vi "Agilent SNA Set Stimulus.vi"(5 "Stimulus":T4={"Use Instrument Settings"=FALSE, "Blank Frequencies"=FALSE, "Sweep Type"=enum."Linear", "Sweep"={"Fstart"=500.0, "Fstop"=1500.0, "Units"=enum."MHz", "Points"=201}, "Power (dBm)"=999.0, "IFBW (Hz)"=-1.0, "Sweep Time (s)"=-1.0, "Calibration"={"State"=FALSE, "String"=""}} {"Sweep Time (s)" format="%.3g"}, 6 "Set Stimulus? (T)":bool=TRUE, 7 "Agilent SNA":T7, 8 "error in (no error)":errorcluster, 9 "Channel":i8=1 min=1 max=99 step=1, 10 "Sorted Measurements":cluster{"Measurements":T1[]}[](array[cluster]) {"Measurements"."Traces"."Parameter"."Stimulus Port" min=1 step=1; "Measurements"."Traces"."Parameter"."Response Port" min=1 step=1}, 11 "VISA Resource Names":T3) -> (0 "error out":errorcluster {"code" format="%.0x"}, 3 "dup VISA Resource Names":T3)   [LabVIEW 2011]
uses:
  TypeDefs/Agilent SNA VISA.ctl
  TypeDefs/Agilent SNA Instrument Info.ctl
  tests/S Parameter/TypeDefs/SP Stimulus Parameters.ctl
  tests/S Parameter/TypeDefs/SP Frequency Units.ctl
  tests/S Parameter/TypeDefs/SP Calibration State.ctl
  TypeDefs/Agilent SNA Measurements.ctl
  tests/S Parameter/TypeDefs/SP Parameter.ctl
  TypeDefs/Agilent SNA Measurement.ctl
  TypeDefs/Agilent SNA Message Mode.ctl
  TypeDefs/Agilent SNA External Trigger Mode.ctl
  TypeDefs/Agilent SNA Sweep Type.ctl
  TypeDefs/Agilent SNA Trigger Mode.ctl
panel:
  in  "Case Constant\n(See Context Help)":bool
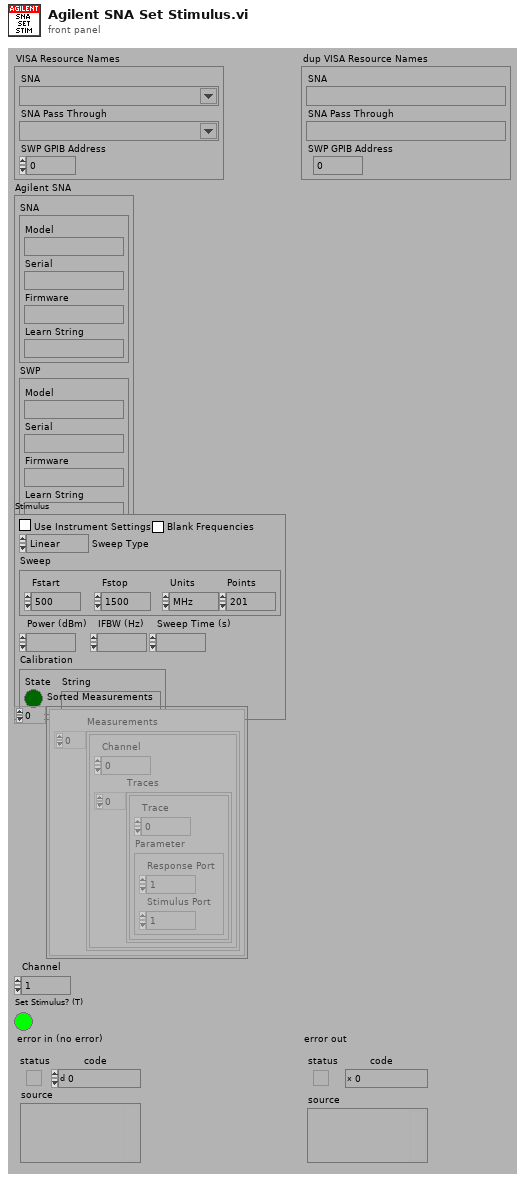
[diagram p1: front panel]
types:
  T1 = typedef "Agilent SNA Measurements.ctl" = cluster{"Channel":i8, "Traces":cluster{"Trace":i8, "Parameter":T2}[]}
  T2 = typedef "SP Parameter.ctl" = cluster{"Stimulus Port":i8, "Response Port":i8}
  T3 = typedef "Agilent SNA VISA.ctl" = cluster{"SNA":refnum<visa-resource-name>, "SNA Pass Through":refnum<visa-resource-name>, "SWP GPIB Address":i32}
  T4 = typedef "SP Stimulus Parameters.ctl" = cluster{"Use Instrument Settings":bool, "Blank Frequencies":bool, "Sweep Type":enum32{"Linear", "Logarithmic", "List", "Power", "CW"}, "Sweep":cluster{"Fstart":dbl, "Fstop":dbl, "Units":T5, "Points":i32}, "Power (dBm)":dbl, "IFBW (Hz)":dbl, "Sweep Time (s)":dbl, "Calibration":T6}
  T5 = typedef "SP Frequency Units.ctl" = enum16{"Hz", "kHz", "MHz", "GHz", "Points"}
  T6 = typedef "SP Calibration State.ctl" = cluster{"State":bool, "String":string}
  T7 = typedef "Agilent SNA Instrument Info.ctl" = cluster{"SNA":cluster{"Model":string, "Serial":string, "Firmware":string, "Learn String":string}, "SWP":cluster{"Model":string, "Serial":string, "Firmware":string, "Learn String":string}}
  T8 = typedef "Agilent SNA Message Mode.ctl" = enum16{"On", "Off"}
  T9 = typedef "Agilent SNA Measurement.ctl" = enum32{"SXX", "A", "B", "C", "R", "A/B", "A/C", "A/R", "B/A", "B/C", "B/R", "C/A", "C/B", "C/R", "R/A", "R/B", "R/C", "Analog In - Aux In"}
  T10 = typedef "Agilent SNA External Trigger Mode.ctl" = enum16{"Internal", "External", "Single/Bus"}
  T11 = typedef "Agilent SNA Sweep Type.ctl" = enum32{"Linear Sweep", "CW Time Sweep", "Frequency List"}
  T12 = typedef "Agilent SNA Trigger Mode.ctl" = enum16{"Continuous", "Hold", "Single"}
  T13 = enum32{"Linear", "Logarithmic", "List", "Power", "CW"}
  T14 = cluster{"Converted Frequency":dbl, "Converted Frequency":dbl}
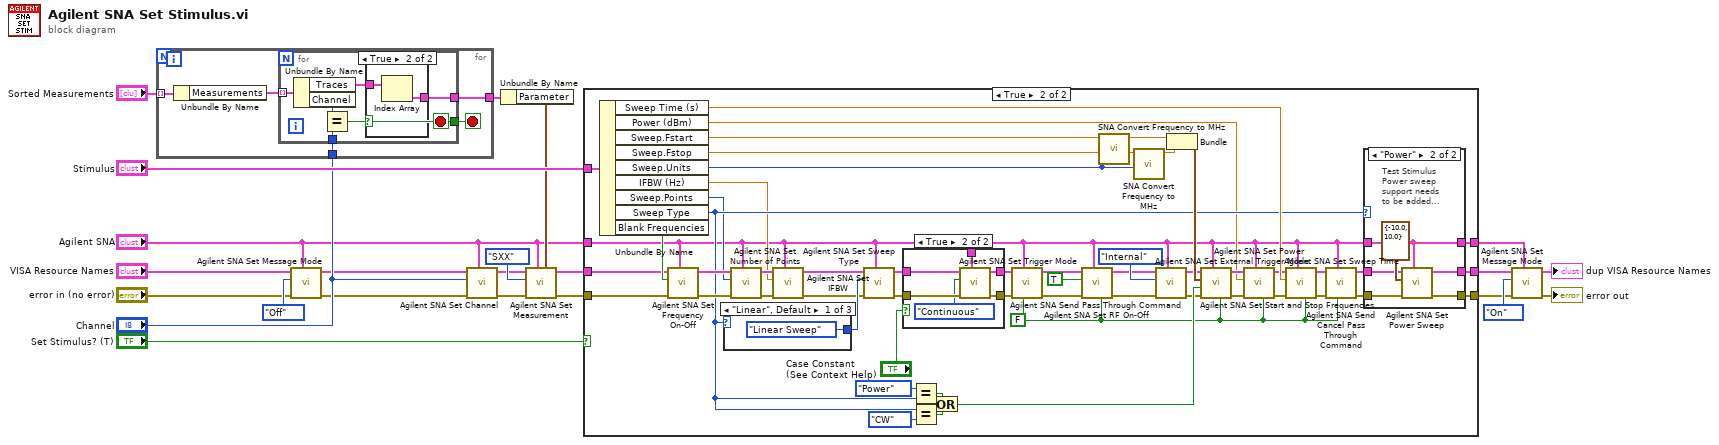
[diagram p0: block diagram]
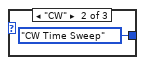
[diagram p4: hidden frame]
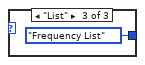
[diagram p5: hidden frame]
diagram:
  n1 = for {
    tunnel: "Sorted Measurements" -> [w28] mode=indexing
    tunnel: "Channel" -> [w26]
    tunnel: [w25] -> w14
    stop <- w24 stop-if-true
    n2 = Unbundle By Name(w28) -> ("Measurements"=w27:T1[])
    n3 = for {
      tunnel: w27 -> [w34] mode=indexing
      tunnel: w26 -> [w31]
      tunnel: [w30] -> w25
      tunnel: [w29] -> w24
      stop <- w29 stop-if-true
      n4 = Unbundle By Name(w34) -> ("Traces"=w32:cluster{"Trace":i8, "Parameter":T2}[], "Channel"=w33:i8)
      n5 = Equal?(x=w33, y=w31) -> (x = y?=w29:bool)
      n6 = case shown="True" w29 {
        tunnel: w32 -> [_ w36]
        tunnel: [_ w35] -> w30
        frame False {
        }
        frame True {
          n7 = Index Array(array=w36) -> (element=w35:cluster{"Trace":i8, "Parameter":T2})  [unwired: 1 in]
        }
      }
    }
  }
  n8 = call "Agilent SNA Set Message Mode.vi"("Agilent SNA & SWP"="Agilent SNA", "error in (no error)"="error in (no error)", "Message Mode"=Agilent_SNA_Message_Mode."Off", "VISA Resource Names"="VISA Resource Names") -> ("error out"=w3:errorcluster, "dup VISA Resource Names"=w4:T3)  [unwired: 6 out]
  n9 = call "Agilent SNA Set Channel.vi"("Agilent SNA & SWP"="Agilent SNA", "error in (no error)"=w3, "Channel"="Channel", "VISA Resource Names"=w4) -> ("error out"=w19:errorcluster, "dup VISA Resource Names"=w20:T3)  [unwired: 6 out]
  n10 = Unbundle By Name(w14) -> ("Parameter"=w13:T2)
  n11 = call "Agilent SNA Set Measurement.vi"("Parameter"=w13, "Agilent SNA & SWP"="Agilent SNA", "error in (no error)"=w19, "Measurement (SXX)"=Agilent_SNA_Measurement."SXX" ("Measurement (S11 - A/R)"), "VISA Resource Names"=w20) -> ("error out"=w18:errorcluster, "dup VISA Resource Names"=w17:T3)  [unwired: 3 in, 2 out]
  n12 = case shown="True" "Set Stimulus? (T)" {
    tunnel: "Stimulus" -> [_ w92]
    tunnel: w18 -> [w39 w76]
    tunnel: w17 -> [w38 w77]
    tunnel: [w39 w63] -> w8
    tunnel: [w38 w64] -> w7
    tunnel: "Agilent SNA" -> [w37 w48]
    tunnel: [w37 w40] -> w1
    frame False {
    }
    frame True {
      w47 = FALSE ("SCPI? (F)")
      n13 = Unbundle By Name(w92) -> ("Sweep Time (s)"=w91:dbl, "Power (dBm)"=w60:dbl, "Sweep.Fstart"=w59:dbl, "Sweep.Fstop"=w58:dbl, "Sweep.Units"=w57:T5, "IFBW (Hz)"=w67:dbl, "Sweep.Points"=w68:i32, "Sweep Type"=w69:T13, "Blank Frequencies"=w83:bool)
      n14 = call "Agilent SNA Set Frequency On-Off.vi"("Agilent SNA & SWP"=w48, "error in (no error)"=w76, "Blank Frequencies (F)"=w83, "VISA Resource Names"=w77) -> ("error out"=w70:errorcluster, "dup VISA Resource Names"=w71:T3)  [unwired: 6 out]
      n15 = case shown="\"Linear\", Default" w69 {
        tunnel: [Agilent_SNA_Sweep_Type."Linear Sweep" ("Sweep Type") Agilent_SNA_Sweep_Type."CW Time Sweep" ("Sweep Type") Agilent_SNA_Sweep_Type."Frequency List" ("Sweep Type")] -> w80
        frame "Linear", Default {
        }
        frame "CW" {
        }
        frame "List" {
        }
      }
      n16 = call "Agilent SNA Set Number of Points.vi"("Agilent SNA & SWP"=w48, "error in (no error)"=w70, "Number Points"=w68, "VISA Resource Names"=w71) -> ("error out"=w74:errorcluster, "dup VISA Resource Names"=w75:T3)  [unwired: 1 in, 5 out]
      n17 = call "Agilent SNA Set IFBW.vi"("Agilent SNA & SWP"=w48, "error in (no error)"=w74, "IFBW, Hz (1000)"=w67, "VISA Resource Names"=w75) -> ("error out"=w73:errorcluster, "dup VISA Resource Names"=w72:T3)  [unwired: 1 in, 5 out]
      n18 = call "Agilent SNA Set Sweep Type.vi"("Agilent SNA & SWP"=w48, "error in (no error)"=w73, "Sweep Type"=w80, "VISA Resource Names"=w72) -> ("error out"=w55:errorcluster, "dup VISA Resource Names"=w56:T3)  [unwired: 1 in, 5 out]
      n19 = case shown="True" "Case Constant\n(See Context Help)" {
        tunnel: [w97 w100] -> w45
        tunnel: [w96 w101] -> w46
        tunnel: w55 -> [w97 w103]
        tunnel: w56 -> [w96 w102]
        tunnel: w48 -> [_ w98]
        frame False {
        }
        frame True {
          n20 = call "Agilent SNA Set Trigger Mode.vi"("Agilent SNA & SWP"=w98, "error in (no error)"=w103, "Trigger Mode"=Agilent_SNA_Trigger_Mode."Continuous", "VISA Resource Names"=w102) -> ("error out"=w100:errorcluster, "dup VISA Resource Names"=w101:T3)  [unwired: 1 in, 5 out]
        }
      }
      n21 = Equal?(x=enum32{"Linear", "Log", "List", "Power", "CW"}."Power" ("Sweep Type"), y=w69) -> (x = y?=w88:bool)
      n22 = Equal?(x=w69, y=enum32{"Linear", "Log", "List", "Power", "CW"}."CW" ("Sweep Type")) -> (x = y?=w87:bool)
      n23 = Or(x=w88, y=w87) -> (x .or. y?=w84:bool)
      n24 = call "Agilent SNA Send Pass Through Command.vi"("SCPI? (F)"=w47, "Agilent SNA & SWP"=w48, "error in (no error)"=w45, "VISA Resource Names"=w46) -> ("error out"=w54:errorcluster, "dup VISA Resource Names"=w53:T3)  [unwired: 6 out]
      n25 = call "Agilent SNA Set RF On-Off.vi"("Passthrough (T)"=w47, "Agilent SNA & SWP"=w48, "error in (no error)"=w54, "RF On (T)"=TRUE, "VISA Resource Names"=w53) -> ("error out"=w41:errorcluster, "dup VISA Resource Names"=w42:T3)  [unwired: 5 out]
      n26 = call "SNA Convert Frequency to MHz.vi"("Units"=w57, "Frequency"=w59) -> ("Converted Frequency"=w82:dbl)  [unwired: 9 out]
      n27 = call "SNA Convert Frequency to MHz.vi"("Units"=w57, "Frequency"=w58) -> ("Converted Frequency"=w81:dbl)  [unwired: 9 out]
      n28 = call "Agilent SNA Set External Trigger Mode.vi"("Agilent SNA & SWP"=w48, "error in (no error)"=w41, "Ext. Trigger Mode"=Agilent_SNA_External_Trigger_Mode."Internal", "VISA Resource Names"=w42) -> ("error out"=w44:errorcluster, "dup VISA Resource Names"=w43:T3)  [unwired: 1 in, 5 out]
      n29 = Bundle("Converted Frequency"=w82, "Converted Frequency"=w81) -> (w89:T14)  [unwired: 1 out]
      n30 = call "Agilent SNA Set Start and Stop Frequencies.vi"("Passthrough (T)"=w47, "Agilent SNA & SWP"=w48, "error in (no error)"=w44, "CW? (f)"=w84, "Start/Stop Freqs, MHz"=w89, "VISA Resource Names"=w43) -> ("error out"=w62:errorcluster, "dup VISA Resource Names"=w61:T3)  [unwired: 1 in, 3 out]
      n31 = call "Agilent SNA Set Power.vi"("Passthrough (T)"=w47, "Agilent SNA & SWP"=w48, "error in (no error)"=w62, "Source Power, dBm (0.0)"=w60, "VISA Resource Names"=w61) -> ("error out"=w65:errorcluster, "dup VISA Resource Names"=w66:T3)  [unwired: 1 in, 4 out]
      n32 = call "Agilent SNA Set Sweep Time.vi"("Passthrough (T)"=w47, "Agilent SNA & SWP"=w48, "error in (no error)"=w65, "Sweep Time, s (-1: Auto)"=w91, "VISA Resource Names"=w66) -> ("error out"=w51:errorcluster, "dup VISA Resource Names"=w52:T3)  [unwired: 1 in, 4 out]
      n33 = call "Agilent SNA Send Cancel Pass Through Command.vi"("SCPI? (F)"=w47, "Agilent SNA & SWP"=w48, "error in (no error)"=w51, "VISA Resource Names"=w52) -> ("error out"=w50:errorcluster, "dup VISA Resource Names"=w49:T3)  [unwired: 6 out]
      n34 = case shown="\"Power\"" w69 {
        tunnel: w50 -> [w106 w109]
        tunnel: w49 -> [w105 w108]
        tunnel: [w105 w111] -> w64
        tunnel: [w106 w110] -> w63
        tunnel: w48 -> [w104 w107]
        tunnel: [w104 w107] -> w40
        frame "Linear", "Logarithmic", "CW", Default {
        }
        frame "Power" {
          # "Test Stimulus\nPower sweep\nsupport needs\nto be added..."
          n35 = call "Agilent SNA Set Power Sweep.vi"("Agilent SNA & SWP"=w107, "error in (no error)"=w109, "Start/Stop Power, dBm"=cluster{"Pstart":dbl, "Pstop":dbl} {"Pstart"=-10.0, "Pstop"=10.0}, "VISA Resource Names"=w108) -> ("error out"=w110:errorcluster, "dup VISA Resource Names"=w111:T3)  [unwired: 6 out]
        }
      }
    }
  }
  n36 = call "Agilent SNA Set Message Mode.vi"("Agilent SNA & SWP"=w1, "error in (no error)"=w8, "Message Mode"=Agilent_SNA_Message_Mode."On", "VISA Resource Names"=w7) -> ("error out"=→"error out":errorcluster, "dup VISA Resource Names"=→"dup VISA Resource Names":T3)  [unwired: 6 out]
